vi "auto loader.vi"(11 "balls":dbl=-1.95) -> ()   [LabVIEW 2019]
uses:
  <vilib>/Rock Robotics/WPI/ThirdParty/Phoenix-LabVIEW/Motor Controller/Controls/CTRE_Phoenix_MotorControl_ControlMode.ctl
  <vilib>/Rock Robotics/WPI/ThirdParty/Phoenix-LabVIEW/Motor Controller/Get/CTRE_Phoenix_MotorController_GetSelectedSensorData.vi
panel:
  in  "rotations":dbl=-1.95
  in  "Cruise Velocity":i32=20000
  in  "Acceleration":i32=20000
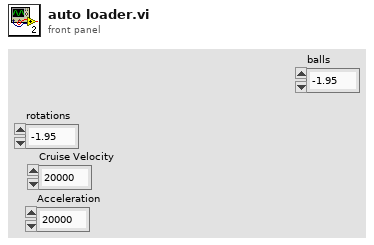
[diagram p1: front panel]
types:
  T1 = typedef "WPI_MotorControlDeviceRef.ctl" = cluster{"DeviceStatus":errorcluster, "Type":T2, "PWM":cluster{"PWM Channel":T3, "DeadBand":T4}, "CAN":cluster{"Device Number":u8, "SetOutput VI Ref":variant, "GetOutput VI Ref":variant, "Enable VI Ref":variant, "Disable VI Ref":variant, "Data":variant}, "Invert":bool, "DIO PWM":cluster{"PWM \"Enable\" Channel":T3, "DIOChannel":T5, "PWM Rate":dbl}}
  T2 = typedef "WPI_MotorControlType.ctl" = enum16{"PWM", "CAN", "DIO PWM"}
  T3 = typedef "FPGA_DIOPWMChannel.ctl" = enum8{"PWM 0", "PWM 1", "PWM 2", "PWM 3", "PWM 4", "PWM 5", "PWM 6", "PWM 7", "PWM 8", "PWM 9", "PWM MXP 0", "PWM MXP 1", "PWM MXP 2", "PWM MXP 3", "PWM MXP 4", "PWM MXP 5", "PWM MXP 6", "PWM MXP 7", "PWM MXP 8", "PWM MXP 9", "Invalid"}
  T4 = typedef "WPI_PWMDeadband.ctl" = cluster{"Name":string, "maxPositivePwm":i32, "minPositivePwm":i32, "centerPwm":i32, "maxNegativePwm":i32, "minNegativePwm":i32, "angularRange":u16}
  T5 = typedef "FPGA_DIOChannel.ctl" = enum8{"DIO 0", "DIO 1", "DIO 2", "DIO 3", "DIO 4", "DIO 5", "DIO 6", "DIO 7", "DIO 8", "DIO 9", "DIO MXP 0", "DIO MXP 1", "DIO MXP 2", "DIO MXP 3", "DIO MXP 4", "DIO MXP 5", "DIO MXP 6", "DIO MXP 7", "DIO MXP 8", "DIO MXP 9", "DIO MXP 10", "DIO MXP 11", "DIO MXP 12", "DIO MXP 13", "DIO MXP 14", "DIO MXP 15", "SPI Port CS1", "SPI Port CS2", "SPI Port CS3", "SPI Port MISO", "SPI Port MOSI", "Invalid"}
  T6 = typedef "CTRE_Phoenix_MotorControl_ControlMode.ctl" = u16
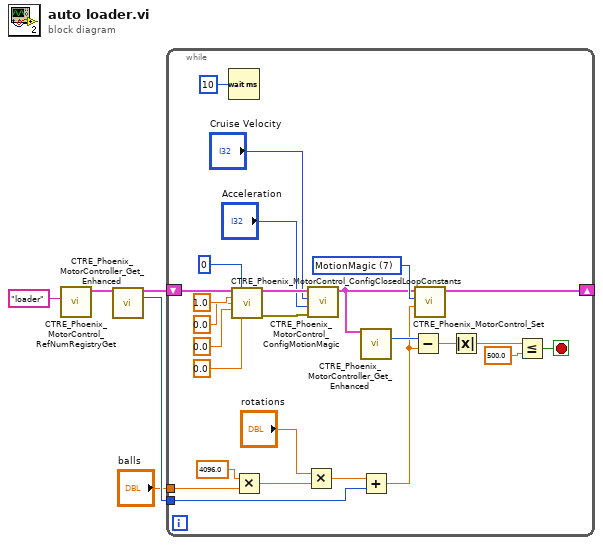
[diagram p0: block diagram]
diagram:
  n1 = call <vilib>:"CTRE_Phoenix_MotorControl_RefNumRegistryGet.vi"("refnum name"="loader") -> ("PhoenixMotorControlDevRef"=w1:T1)  [unwired: 9 in, 1 out]
  n2 = call-poly <vilib>:"CTRE_Phoenix_MotorController_Get_Enhanced.vi"("PhoenixMotorControlDevRef"=w1) -> ("PhoenixMotorControlDevRef"=w5:T1, "Position (Raw Sensor Units)"=w4:i32)  [unwired: 11 in, 2 out]
  n3 = while {
    shift-right: [w30] -> _
    shift-left: w5 -> [w12]
    tunnel: w4 -> [w20]
    tunnel: "balls" -> [w8]
    stop <- w25 stop-if-true
    w31 = T6 7 items=["PercentOutput"=0, "Position"=1, "Velocity"=2, "Current"=3, "Follower"=5, "MotionProfile"=6, "MotionMagic"=7, "MotionProfileArc"=10, "Disabled"=15] ("Control Mode")
    n4 = Wait (ms)(milliseconds to wait=u32 10) -> ()  [unwired: 1 out]
    n5 = call <vilib>:"CTRE_Phoenix_MotorControl_ConfigClosedLoopConstants.vi"("PhoenixMotorControlDevRef"=w12, "slotIdx"=0, "P"=1.0, "I"=0.0, "D"=0.0, "F"=0.0) -> ("PhoenixMotorControlDevRef"=w14:T1, "error out"=w13:errorcluster)  [unwired: 8 in]
    n6 = Multiply(x=4096.0 ("y"), y=w8) -> (x*y=w7:dbl)
    n7 = Multiply(x="rotations", y=w7) -> (x*y=w22:dbl)
    n8 = call <vilib>:"CTRE_Phoenix_MotorControl_ConfigMotionMagic.vi"("error in (no error)"=w13, "Acceleration"="Acceleration", "Cruise Velocity"="Cruise Velocity", "PhoenixMotorControlDevRef"=w14) -> ("PhoenixMotorControlDevRef"=w11:T1)  [unwired: 6 in, 1 out]
    n9 = call-poly <vilib>:"CTRE_Phoenix_MotorController_Get_Enhanced.vi"("PhoenixMotorControlDevRef"=w11) -> ("Position (Raw Sensor Units)"=w27:i32)  [unwired: 11 in, 3 out]
    n10 = Add(x=w22, y=w20) -> (x+y=w21:dbl)
    n11 = Subtract(x=w27, y=w21) -> (x-y=w24:dbl)
    n12 = call <vilib>:"CTRE_Phoenix_MotorControl_Set.vi"("Output"=w21, "Control Mode"=w31, "PhoenixMotorControlDevRef"=w11) -> ("PhoenixMotorControlDevRef"=w30:T1)  [unwired: 7 in, 1 out]
    n13 = Absolute Value(x=w24) -> (abs(x)=w26:dbl)
    n14 = Less Or Equal?(x=w26, y=500.0) -> (x <= y?=w25:bool)
  }
